vi "TW_ReadData.vi"(11 "Property":string) -> (2 "value":string)   [LabVIEW 2019]
panel:
  out "Comm":T1
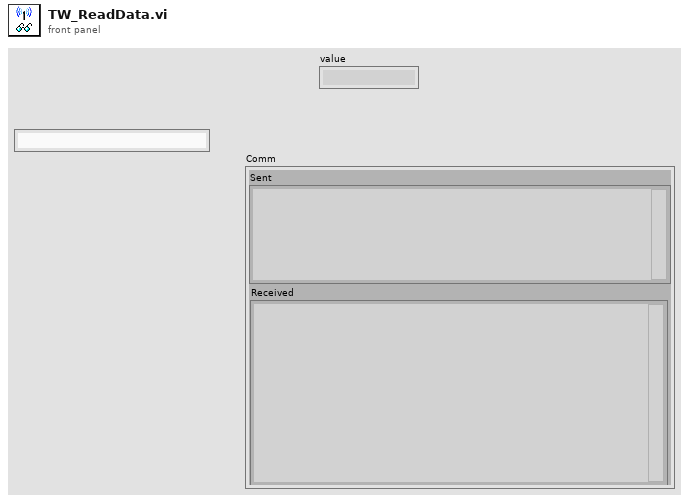
[diagram p1: front panel]
types:
  T1 = cluster{"url":string, "sent headers":string, "sent body":string, "headers":string, "body":string, "Sent":string, "Received":string}
  T2 = enum16{"GET", "PUT", "POST", "MultiPOST", "DELETE"}
  T3 = cluster{"Name":string, "BaseURL":string, "AppKey":string, "Headers":string[], "Timeout":i32}
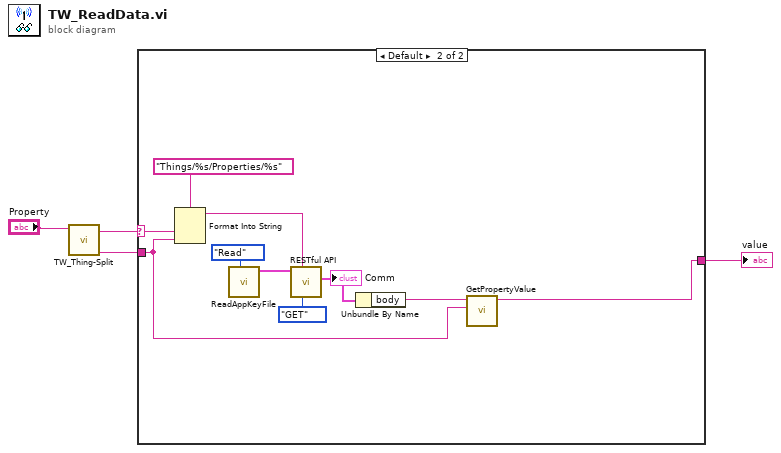
[diagram p0: block diagram]
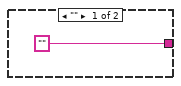
[diagram p2: hidden frame]
diagram:
  n1 = call "TW_Thing-Split.vi"("Property"="Property") -> ("Property"=w1:string, "Thing"=w2:string)  [unwired: 9 in]
  n2 = case shown="Default" w2 {
    selector: w2 -> [_ w10]
    tunnel: ["" ("body") w7] -> w4
    tunnel: w1 -> [_ w6]
    frame "" {
    }
    frame Default {
      n3 = Format Into String(format string="Things/%s/Properties/%s" ("url"), w10, w6) -> (resulting string=w15:string)  [unwired: 2 in, 1 out]
      n4 = call "ReadAppKeyFile.vi"("Task"=enum16{"Read", "Write"}."Read") -> ("Device Out"=w14:T3)  [unwired: 8 in, 2 out]
      n5 = call "RESTful API.vi"("Method"=T2."GET", "url"=w15, "Device In"=w14) -> ("Comm"=w9:T1)  [unwired: 6 in, 2 out]
      "Comm" <- w9
      n6 = Unbundle By Name(w9) -> ("body"=w8:string)
      n7 = call "GetPropertyValue.vi"("Property"=w6, "body"=w8) -> ("String out"=w7:string)  [unwired: 9 in]
    }
  }
  "value" <- w4
